vi "testQuerySystemDefinitionFile.vi"(8 "error in (no error)":errorcluster, 11 "TestCase in":refnum<class "VeriStandTestUtilitiesUnitTests.lvclass">) -> (0 "error out":errorcluster, 3 "TestCase out":refnum<class "VeriStandTestUtilitiesUnitTests.lvclass">)   [LabVIEW 2015, in "VeriStandTestUtilitiesUnitTests.lvclass"]
uses:
  VeriStandTestUtilitiesUnitTests.lvclass
  TargetInformation.ctl
  <vilib>/addons/_JKI Toolkits/VI Tester/TestCase.llb/TestCase.lvclass
  VeriStandTestUtilities.lvlib
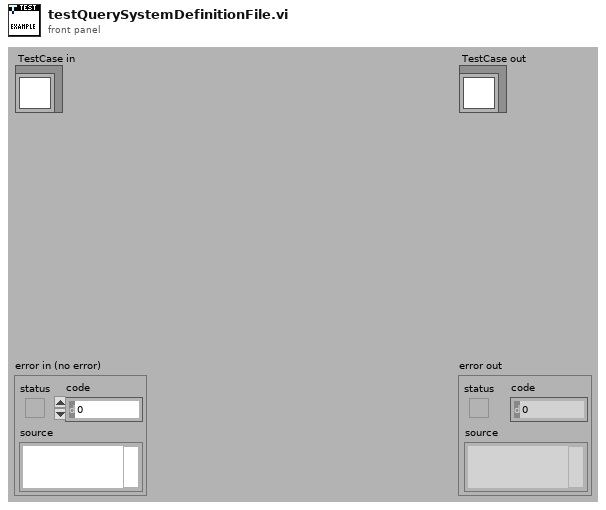
[diagram p1: front panel]
types:
  T1 = typedef "VeriStandTestUtilities.lvlib/TargetInformation.ctl" = cluster{"Name":string, "IP Address":string, "Operating System":string, "Target Rate":dbl, "Chassis List":cluster{"Name":string, "Devices":string[]}[], "Custom Device List":string[]}
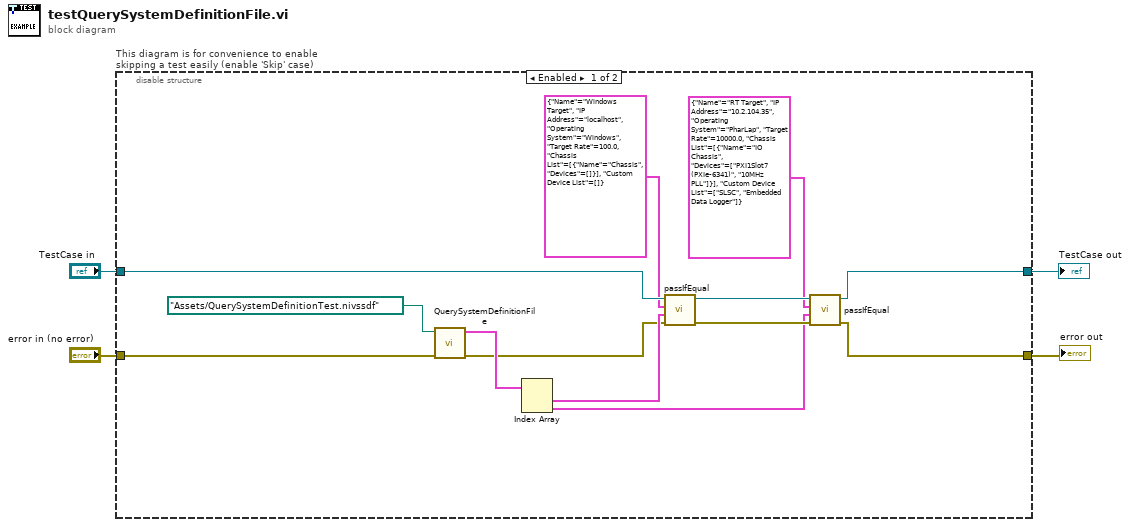
[diagram p0: block diagram]
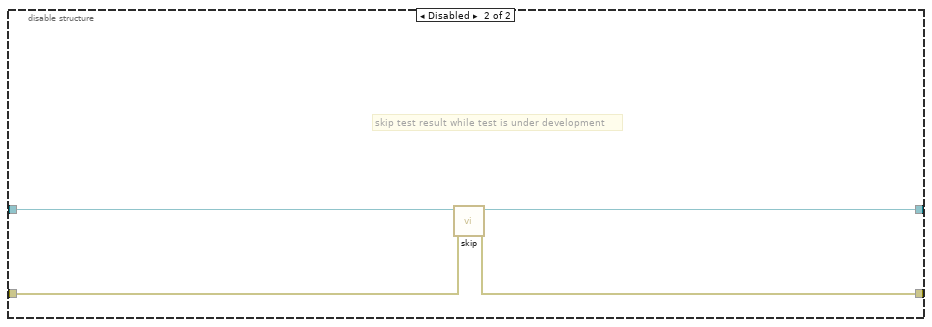
[diagram p2: hidden frame]
diagram:
  n1 = disable-structure "This diagram is for convenience to enable skipping a test easily (enable 'Skip' case)" shown="Enabled" {
    disable-tunnel: "TestCase in" -> [w14 w21]
    disable-tunnel: [w5 w19] -> w1
    disable-tunnel: [w8 w20] -> w3
    disable-tunnel: "error in (no error)" -> [w17 w18]
    frame Enabled {
      n2 = call "QuerySystemDefinitionFile.vi"("error in (no error)"=w17, "Absolute System Definiton File in"=path "Assets/QuerySystemDefinitionTest.nivssdf" ("custom device xml path")) -> ("error out"=w11:errorcluster, "Target Information List out"=w15:T1[])  [unwired: 8 in]
      n3 = Index Array(array=w15) -> (element #1=w12:T1, element #2=w6:T1)  [unwired: 2 in]
      n4 = call-dynamic "passIfEqual.vi"("error in (no error)"=w11, "y"=w12, "x"=T1 {"Name"="Windows Target", "IP Address"="localhost", "Operating System"="Windows", "Target Rate"=100.0, "Chassis List"=[{"Name"="Chassis", "Devices"=[]}], "Custom Device List"=[]} ("element"), "TestCase in"=w14) -> ("error out"=w9:errorcluster, "TestCase out"=w10:refnum<class "VeriStandTestUtilitiesUnitTests.lvclass">)  [unwired: 6 in]
      n5 = call-dynamic "passIfEqual.vi"("error in (no error)"=w9, "y"=w6, "x"=T1 {"Name"="RT Target", "IP Address"="10.2.104.35", "Operating System"="PharLap", "Target Rate"=10000.0, "Chassis List"=[{"Name"="IO Chassis", "Devices"=["PXI1Slot7 (PXIe-6341)", "10MHz PLL"]}], "Custom Device List"=["SLSC", "Embedded Data Logger"]} ("element 2"), "TestCase in"=w10) -> ("error out"=w8:errorcluster, "TestCase out"=w5:refnum<class "VeriStandTestUtilitiesUnitTests.lvclass">)  [unwired: 6 in]
    }
    frame Disabled {
      # "skip test result while test is under development"
      n6 = call <vilib>:"skip.vi"("error in (no error)"=w18, "TestCase in"=w21) -> ("error out"=w20:errorcluster, "TestCase out"=w19:refnum<class "VeriStandTestUtilitiesUnitTests.lvclass">)  [unwired: 8 in]
    }
  }
  "error out" <- w3
  "TestCase out" <- w1
